vi "inteference V2.vi"(7 "number of points":i32, 8 "complex region":T1={"max re"=5.161869466666667e-06, "min re"=5.176843333333334e-06, "max im"=-2.467216e-05, "min im"=-0.001573233, "delta re"=0.003211203, "delta im"=0.00165815, "center re"=0.0015485608400000002, "delta  z"=0.0015530530000000002+0.0i, "center im"=0.0, "center z"=0.0+0.0i, "d im"=0.0, "d re"=0.0, "d z"=0.0+0.0i}, 9 "pond":cdb[][](array[numeric]), 10 "point sources":cdb[](array[numeric]), 11 "wave packet":cdb[][](array[numeric])) -> (3 "pond out":cdb[][](array[numeric]))   [LabVIEW 2010]
uses:
  complex region.ctl
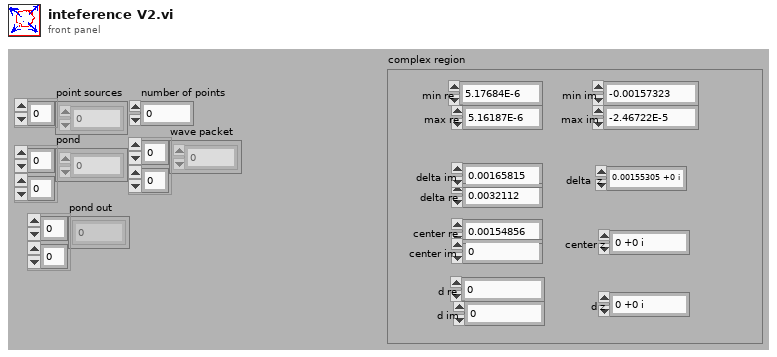
[diagram p1: front panel]
types:
  T1 = typedef "complex region.ctl" = cluster{"max re":dbl, "min re":dbl, "max im":dbl, "min im":dbl, "delta re":dbl, "delta im":dbl, "center re":dbl, "delta  z":cdb, "center im":dbl, "center z":cdb, "d im":dbl, "d re":dbl, "d z":cdb}
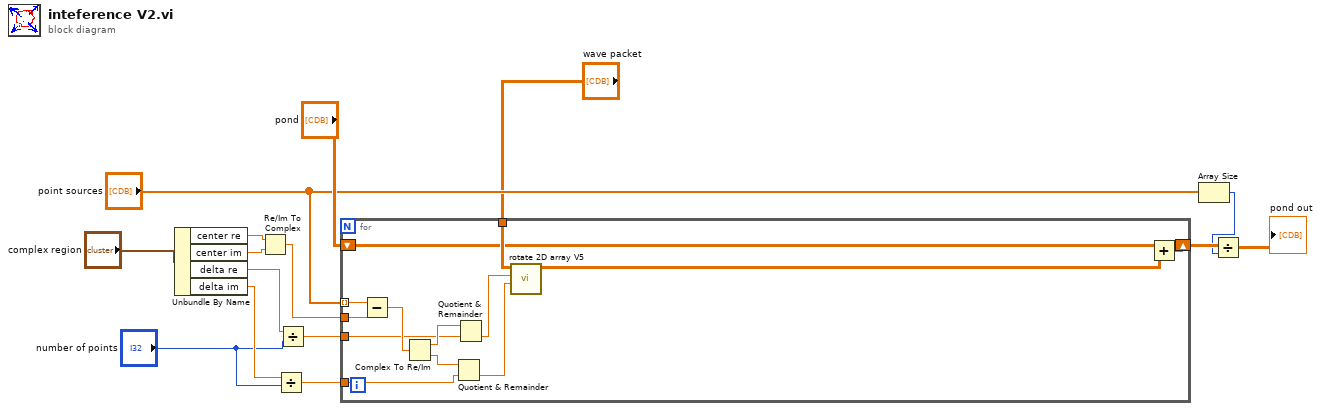
[diagram p0: block diagram]
diagram:
  n1 = Unbundle By Name("complex region") -> ("center re"=w15:dbl, "center im"=w14:dbl, "delta re"=w5:dbl, "delta im"=w4:dbl)
  n2 = Re/Im To Complex(1:w14, 2:w15) -> (0:w13:cdb)
  n3 = Divide(x=w4, y="number of points") -> (x/y=w1:dbl)
  n4 = Divide(x=w5, y="number of points") -> (x/y=w2:dbl)
  n5 = for {
    shift-right: [w25] -> w12
    shift-left: "pond" -> [w27]
    tunnel: "point sources" -> [w24] mode=indexing
    tunnel: "wave packet" -> [w28]
    tunnel: w13 -> [w23]
    tunnel: w2 -> [w20]
    tunnel: w1 -> [w18]
    n6 = Subtract(x=w24, y=w23) -> (x-y=w22:cdb)
    n7 = Complex To Re/Im(x + iy=w22) -> (x=w21:dbl, y=w19:dbl)
    n8 = Quotient & Remainder(x=w19, y=w18) -> (floor(x/y)=w16:dbl)  [unwired: 1 out]
    n9 = Quotient & Remainder(x=w21, y=w20) -> (floor(x/y)=w17:dbl)  [unwired: 1 out]
    n10 = call "rotate 2D array V5.vi"("rotate y"=w16, "rotate x"=w17, "array in"=w28) -> ("array out"=w26:cdb[][])  [unwired: 8 in]
    n11 = Add(x=w27, y=w26) -> (x+y=w25:cdb[][])
  }
  n12 = Array Size(array="point sources") -> (size(s)=w11:i32)
  n13 = Divide(x=w12, y=w11) -> (x/y=→"pond out":cdb[][])
